vi "getFieldIdx.vi"(8 "error in (no error)":errorcluster, 9 "Mapping File Name":string="sensorNameToFieldIdx.txt", 10 "Sensor Name":string[](array[string]), 11 "OptStateEsti in":refnum<class "OptStateEsti.lvclass">) -> (0 "error out":errorcluster, 2 "Field Idx":i32[](array[numeric]), 3 "OptStateEsti out":refnum<class "OptStateEsti.lvclass">)   [LabVIEW 2016, in "OptStateEsti.lvclass"]
doc: "Get the array of field index based on the canonical sensor name (e.g. \"R:2,2 S:1,1\") and mapping file."
uses:
  OptStateEsti.lvclass
  OptStateEsti.lvclass/OptStateEsti.ctl
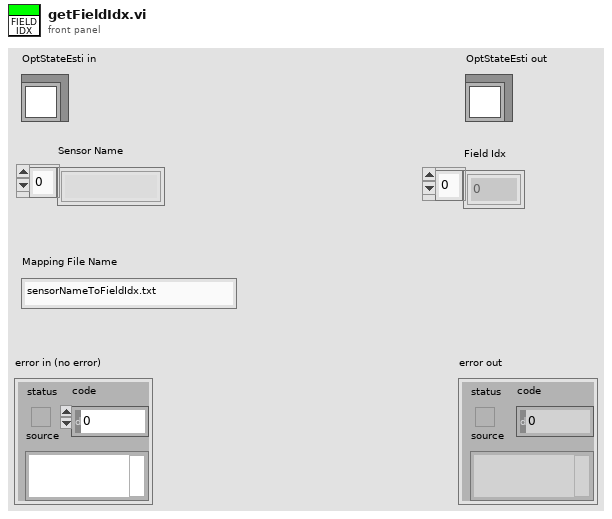
[diagram p1: front panel]
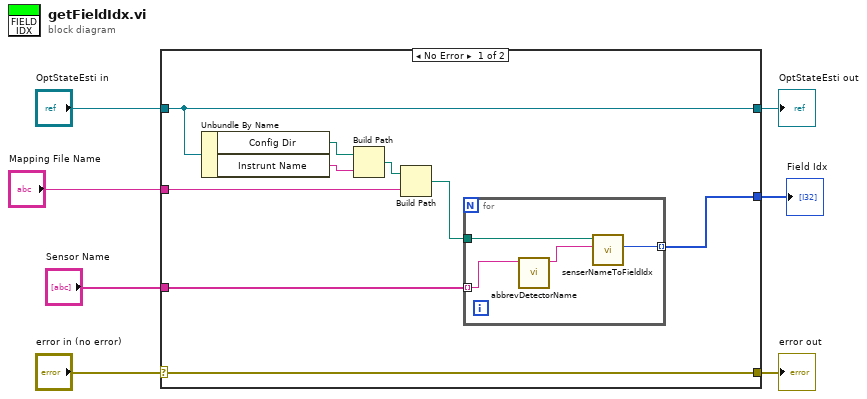
[diagram p0: block diagram]
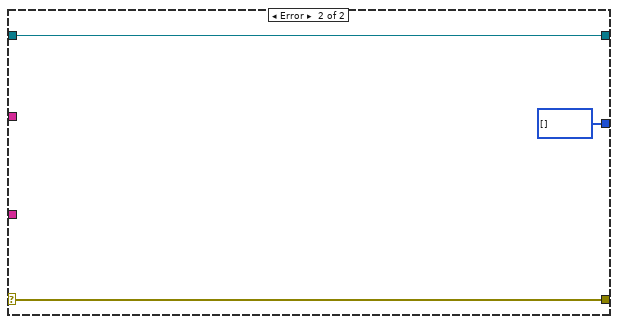
[diagram p2: hidden frame]
diagram:
  n1 = case shown="No Error" "error in (no error)" {
    selector: "error in (no error)" -> [w16 w23]
    tunnel: [w16 w23] -> w6
    tunnel: [w15 w22] -> w4
    tunnel: "OptStateEsti in" -> [w15 w22]
    tunnel: "Mapping File Name" -> [w11 _]
    tunnel: "Sensor Name" -> [w10 _]
    tunnel: [w8 i32[] []] -> w1
    frame No Error {
      n2 = Unbundle By Name(w15) -> ("Config Dir"=w14:path, "Instrunt Name"=w13:string)
      n3 = Build Path(base path=w14, name or relative path=w13) -> (appended path=w12:path)
      n4 = Build Path(base path=w12, name or relative path=w11) -> (appended path=w9:path)
      n5 = for {
        tunnel: w9 -> [w20]
        tunnel: w10 -> [w18] mode=indexing
        tunnel: [w19] -> w8 mode=indexing
        n6 = call "abbrevDetectorName.vi"("Canonical Name"=w18) -> ("Abbreviated Detector Name"=w17:string)  [unwired: 9 in, 1 out]
        n7 = call "senserNameToFieldIdx.vi"("Sensor Name"=w17, "Path"=w20) -> ("Idx of Field"=w19:i32)  [unwired: 8 in, 1 out]
      }
    }
    frame Error {
    }
  }
  "error out" <- w6
  "OptStateEsti out" <- w4
  "Field Idx" <- w1
